vi "Actor Test.vi"() -> ()   [LabVIEW 2020]
uses:
  PPL/HDH.Actor Framework.Core.Publisher.lvlibp/Publisher/Publisher.lvclass
  C:/Current projects/WS/PPL/HDH.Actor Framework.Core.Actor.lvlibp/1abvi3w/vi.lib/ActorFramework/Actor/Actor.lvclass
  Actor/Test Actor/Test Actor.lvclass
  PPL/HDH.Actor Framework.Core.File Writer_TDMS.lvlibp/File Writer_TDMS/File Writer_TDMS.lvclass
  PPL/HDH.Actor Framework.Core.Instrument Handler.lvlibp/Instrument Handler/Instrument Handler.lvclass
  Data/Test Double Data/Test Double Data.lvclass
  C:/Current projects/WS/PPL/HDH.Data.Generic.lvlibp/Data.lvclass
  PPL/HDH.Actor Framework.Core.Data Tracker.lvlibp/Data Tracker/Data Tracker.lvclass
  PPL/HDH.Actor Framework.Core.Actor.lvlibp/1abvi3w/vi.lib/ActorFramework/Message Enqueuer/Message Priority.ctl
  PPL/HDH.Actor Framework.Core.Graph.lvlibp/Graph/Graph.lvclass
  PPL/HDH.Actor Framework.Core.Data Repository.lvlibp/Data Repository/Data Repository.lvclass
  PPL/HDH.Actor Framework.Core.Actor.lvlibp/1abvi3w/vi.lib/ActorFramework/Actor/Actor.lvclass
  PPL/HDH.Actor Framework.Core.Publisher.lvlibp/Publisher Messages/Launch Subscriber Msg/Launch Subscriber Msg.lvclass
  PPL/HDH.Actor Framework.Core.Actor.lvlibp/1abvi3w/vi.lib/ActorFramework/Message Enqueuer/Message Enqueuer.lvclass
  PPL/HDH.Actor Framework.Core.Publisher.lvlibp/Messages/Ping Msg/Ping Msg.lvclass
  PPL/HDH.Actor Framework.Core.Actor.lvlibp/1abvi3w/vi.lib/ActorFramework/Stop Msg/Stop Msg.lvclass
  PPL/HDH.Actor Framework.Core.File Writer.lvlibp/File Writer/File Writer.lvclass
  C:/Current projects/WS/PPL/HDH.Actor Framework.Core.File Writer.lvlibp/File Writer/File Writer.lvclass
  C:/Current projects/WS/PPL/HDH.Actor Framework.Core.Actor.lvlibp/1abvi3w/vi.lib/ActorFramework/Message/Message.lvclass
panel:
  out "error out":errorcluster
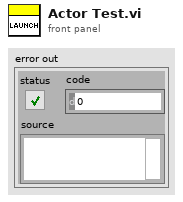
[diagram p1: front panel]
types:
  T1 = typedef "HDH.Actor Framework.Core.Actor.lvlibp/Message Enqueuer.lvclass/Message Priority.ctl" = enum16{"Low", "Normal", "High"}
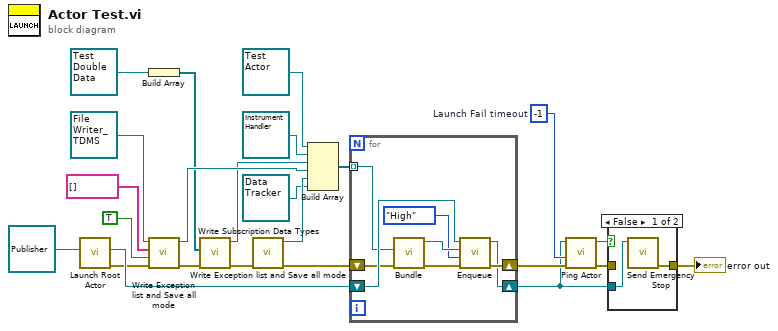
[diagram p0: block diagram]
diagram:
  w22 = -1  # Launch Fail timeout
  n1 = call "Launch Root Actor.vi"("Actor"=refnum<class "Publisher.lvclass"> refnum ("HDH.Actor Framework.Core.Publisher.lvlibp:Publisher.lvclass")) -> ("error out"=w10:errorcluster, "Actor's Enqueuer"=w23:refnum<class "Message Enqueuer.lvclass">)  [unwired: 9 in]
  n2 = Build Array(refnum<class "Test Double Data.lvclass"> refnum ("Test.lvlib:Test Double Data.lvclass")) -> (w7:refnum<class "Test Double Data.lvclass">[])
  n3 = call "Write Exception list and Save all mode.vi"("error in (no error)"=w10, "Save all mode?"=TRUE, "Exception list"=string[] [], "File Writer in"=refnum<class "File Writer_TDMS.lvclass"> refnum ("HDH.Actor Framework.Core.File Writer_TDMS.lvlibp:File Writer_TDMS.lvclass")) -> ("error out"=w5:errorcluster, "File Writer out"=w13:refnum<class "File Writer_TDMS.lvclass">)  [unwired: 6 in]
  n4 = call "Write Subscription Data Types.vi"("error in (no error)"=w5, "Subscription Data Types"=w7) -> ("error out"=w3:errorcluster, "Graph out"=w6:refnum<class "Graph.lvclass">)  [unwired: 8 in]
  n5 = call "Write Exception list and Save all mode.vi"("error in (no error)"=w3) -> ("error out"=w2:errorcluster, "Data Repository out"=w4:refnum<class "Data Repository.lvclass">)  [unwired: 9 in]
  n6 = Build Array(refnum<class "Test Actor.lvclass"> refnum ("Test.lvlib:Test Actor.lvclass"), refnum<class "Instrument Handler.lvclass"> refnum ("HDH.Actor Framework.Core.Instrument Handler.lvlibp:Instrument Handler.lvclass"), w6, w13, w4, refnum<class "Data Tracker.lvclass"> refnum ("HDH.Actor Framework.Core.Data Tracker.lvlibp:Data Tracker.lvclass")) -> (w15:refnum<class "Actor.lvclass">[])
  n7 = for {
    shift-right: [w26] -> w17
    shift-left: w23 -> [w32]
    shift-right: [w27] -> w21
    shift-left: w2 -> [w30]
    tunnel: w15 -> [w25] mode=indexing
    n8 = call "Bundle.vi"("error in (no error)"=w30, "Actor"=w25) -> ("error out"=w29:errorcluster, "Launch Subscriber Msg out"=w31:refnum<class "Launch Subscriber Msg.lvclass">)  [unwired: 8 in]
    n9 = call "Enqueue.vi"("error in (no error)"=w29, "Message Priority (Normal)"=Message_Priority."High", "Message"=w31, "Message Enqueuer in"=w32) -> ("error out"=w27:errorcluster, "Message Enqueuer out"=w26:refnum<class "Message Enqueuer.lvclass">)  [unwired: 6 in]
  }
  n10 = call "Ping Actor.vi"("error in (no error)"=w21, "Timeout if waiting(-1ms)"=w22, "Target Enqueuer"=w17) -> ("error out"=w19:errorcluster, "Success?"=w20:bool)  [unwired: 7 in]
  n11 = case shown="False" w20 {
    tunnel: w19 -> [_ w35]
    tunnel: [w33 w35] -> w18
    tunnel: w17 -> [w34 _]
    frame False {
      n12 = call "Send Emergency Stop.vi"("Message Enqueuer"=w34) -> ("error out"=w33:errorcluster)  [unwired: 10 in]
    }
    frame True {
    }
  }
  "error out" <- w18
